vi "Shooter.vi"   [LabVIEW 2012]
uses:
  Robot Global Data.vi
  ShooterStates.ctl
types:
  T1 = typedef "ShooterStates.ctl" = enum16{"Begin", "Spin Wheel", "Window Motor Spin", "Window Motor Wait", "Window Motor Off", "Finish"}
  T2 = typedef "WPI_MotorControlDeviceRef.ctl" = cluster{"DeviceStatus":errorcluster, "Type":enum16{"PWM", "CAN"}, "PWM":cluster{"Digital Module":T3, "PWM Channel":T4, "DeadBand":T5}, "CAN":cluster{"Device Number":u8, "Control Mode":T6, "Semaphore":T7, "Max Vout":dbl}, "Invert":bool, "TransformRef":T8, "InvTransformRef":T8}
  T3 = typedef "FPGA_TypedefDigitalModule.ctl" = enum16{"Digital Module 1", "Digital Module 2"}
  T4 = typedef "FPGA_DIOPWMChannel.ctl" = enum8{"PWM 1", "PWM 2", "PWM 3", "PWM 4", "PWM 5", "PWM 6", "PWM 7", "PWM 8", "PWM 9", "PWM 10", "Invalid"}
  T5 = typedef "WPI_PWMDeadband.ctl" = cluster{"Name":string, "maxPositivePwm":i32, "minPositivePwm":i32, "centerPwm":i32, "maxNegativePwm":i32, "minNegativePwm":i32, "angularRange":u16}
  T6 = typedef "WPI_CANJaguar_ControlMode.ctl" = enum8{"Percent VBus", "Current", "Speed", "Position", "Voltage"}
  T7 = typedef "Semaphore RefNum" = refnum<k1>
  T8 = typedef "WPI_PWMTransform_ConPane.ctl" = refnum<vi>
  T9 = typedef "WPI_JoystickButtonState.ctl" = cluster{"Button 1":bool, "Button 2":bool, "Button 3":bool, "Button 4":bool, "Button 5":bool, "Button 6":bool, "Button 7":bool, "Button 8":bool, "Button 9":bool, "Button 10":bool, "Button 11":bool, "Button 12":bool}
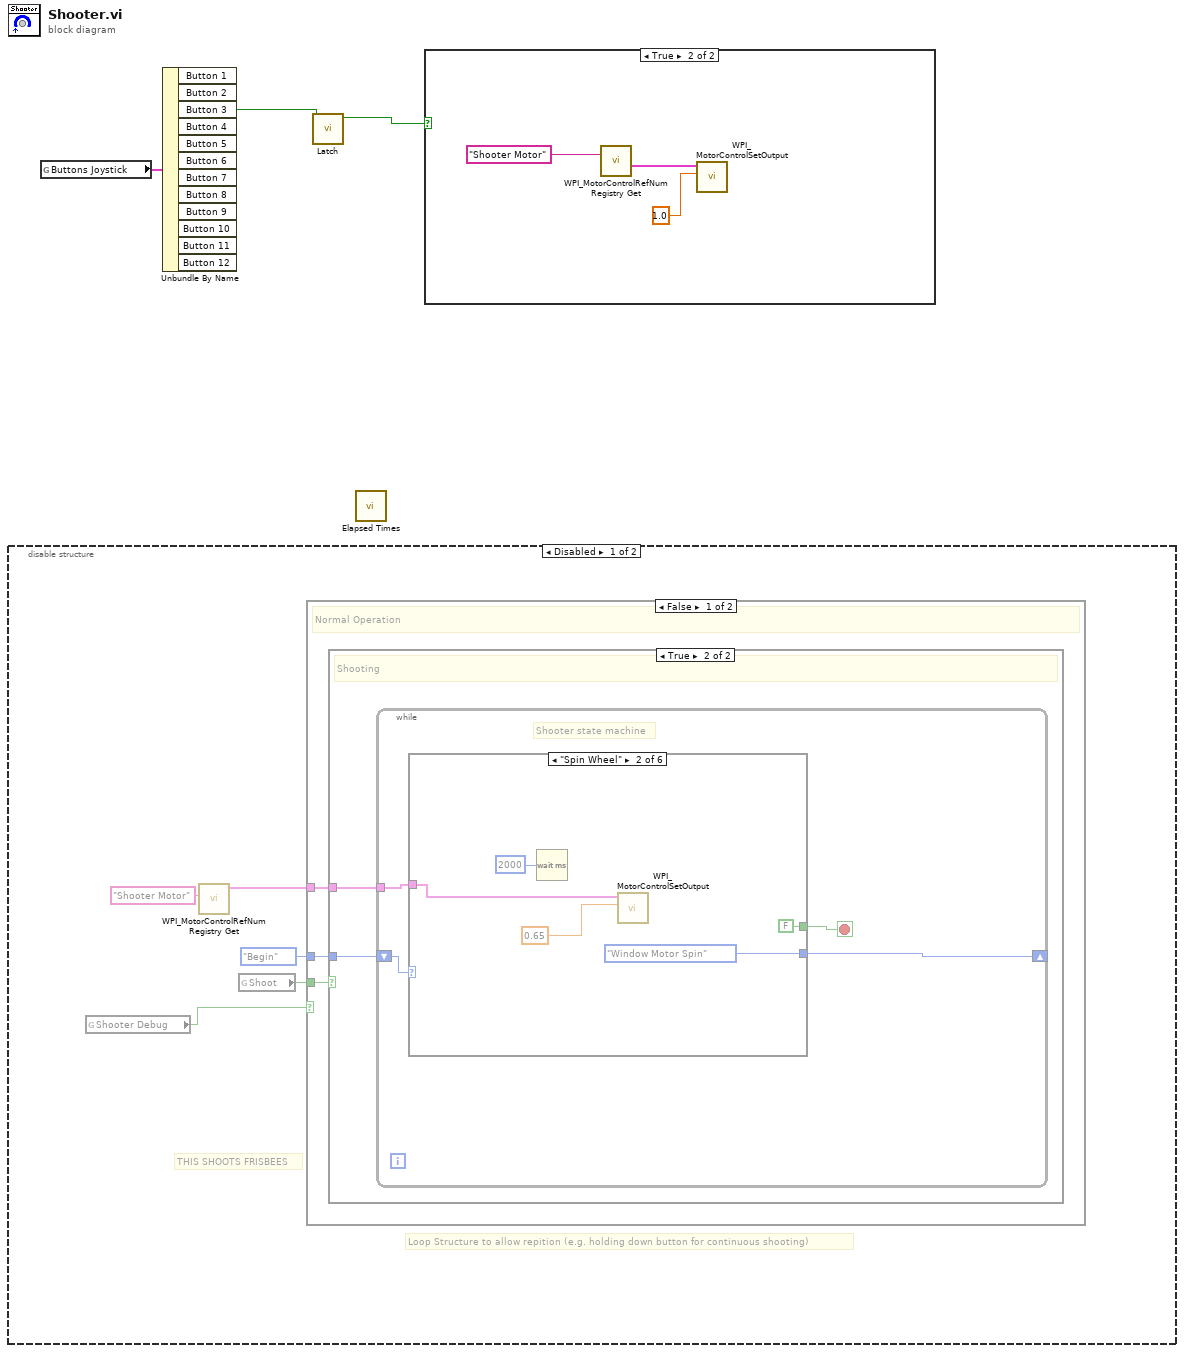
[diagram p0: block diagram]
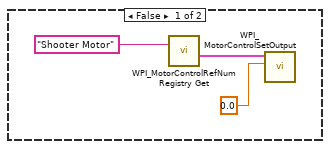
[diagram p2: hidden frame]
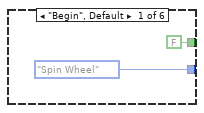
[diagram p4: hidden frame]
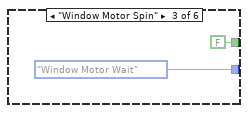
[diagram p5: hidden frame]
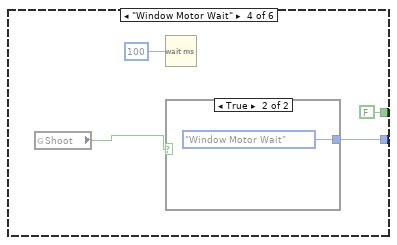
[diagram p6: hidden frame]
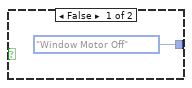
[diagram p7: hidden frame]
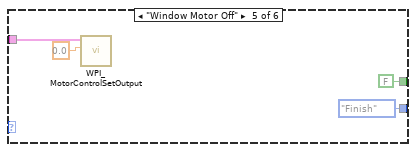
[diagram p8: hidden frame]
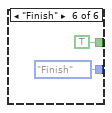
[diagram p9: hidden frame]
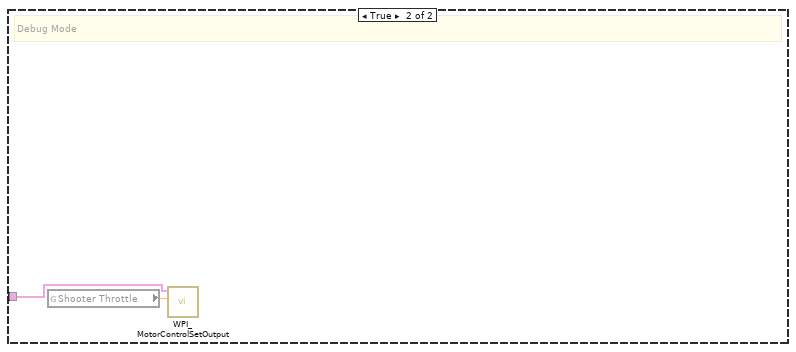
[diagram p10: hidden frame]
diagram:
  n1 = disable-structure shown="Disabled" {
    frame Disabled {
      # "Loop Structure to allow repition (e.g. holding down button for continuous shooting)"
      # "THIS SHOOTS FRISBEES"
      n2 = global read "Robot Global Data.vi" "Shooter Debug"() -> (w4:bool)
      n3 = call <vilib>:"WPI_MotorControlRefNum Registry Get.vi"("refnum name"="Shooter Motor") -> ("MotorControlDevRef"=w5:T2)  [unwired: 9 in, 1 out]
      n4 = global read "Robot Global Data.vi" "Shoot"() -> (w6:bool)
      n5 = case shown="False" w4 {
        tunnel: ShooterStates."Begin" -> [w11 _]
        tunnel: w5 -> [w10 w39]
        tunnel: w6 -> [w9 _]
        frame False {
          # "Normal Operation"
          n6 = case shown="True" w9 {
            tunnel: w11 -> [_ w13]
            tunnel: w10 -> [_ w12]
            frame False {
              # "Not Shooting"
            }
            frame True {
              # "Shooting"
              n7 = while {
                shift-right: [w16] -> _
                shift-left: w13 -> [w17]
                tunnel: w12 -> [w15]
                stop <- w14 stop-if-true
                # "Shooter state machine"
                n8 = case shown="\"Spin Wheel\"" w17 {
                  tunnel: [ShooterStates."Spin Wheel" ShooterStates."Window Motor Spin" ShooterStates."Window Motor Wait" w30 ShooterStates."Finish" ShooterStates."Finish"] -> w16
                  tunnel: w15 -> [_ w21 _ _ w35 _]
                  tunnel: [FALSE FALSE FALSE FALSE FALSE TRUE] -> w14
                  frame "Begin", Default {
                  }
                  frame "Spin Wheel" {
                    n9 = Wait (ms)(milliseconds to wait=u32 2000) -> ()  [unwired: 1 out]
                    n10 = call <vilib>:"WPI_MotorControlSetOutput.vi"("Output"=0.65, "MotorControlDevRef"=w21) -> ()  [unwired: 7 in, 3 out]
                  }
                  frame "Window Motor Spin" {
                  }
                  frame "Window Motor Wait" {
                    n11 = global read "Robot Global Data.vi" "Shoot"() -> (w27:bool)
                    n12 = Wait (ms)(milliseconds to wait=u32 100) -> ()  [unwired: 1 out]
                    n13 = case shown="True" w27 {
                      tunnel: [ShooterStates."Window Motor Off" ShooterStates."Window Motor Wait"] -> w30
                      frame False {
                      }
                      frame True {
                      }
                    }
                  }
                  frame "Window Motor Off" {
                    n14 = call <vilib>:"WPI_MotorControlSetOutput.vi"("Output"=0.0, "MotorControlDevRef"=w35) -> ()  [unwired: 7 in, 3 out]
                  }
                  frame "Finish" {
                  }
                }
              }
            }
          }
        }
        frame True {
          # "Debug Mode"
          n15 = global read "Robot Global Data.vi" "Shooter Throttle"() -> (w40:dbl)
          n16 = call <vilib>:"WPI_MotorControlSetOutput.vi"("Output"=w40, "MotorControlDevRef"=w39) -> ()  [unwired: 7 in, 3 out]
        }
      }
    }
    frame Enabled {
    }
  }
  n17 = global read "Robot Global Data.vi" "Buttons Joystick"() -> (w3:T9)
  n18 = Unbundle By Name(w3) -> ("Button 3"=w2:bool)  [unwired: 11 out]
  n19 = call "Latch.vi"("Input"=w2) -> ("Output"=w1:bool)  [unwired: 9 in]
  n20 = call "Elapsed Times.vi"() -> ()  [unwired: 3 in, 1 out]
  n21 = case shown="True" w1 {
    frame False {
      n22 = call <vilib>:"WPI_MotorControlRefNum Registry Get.vi"("refnum name"="Shooter Motor") -> ("MotorControlDevRef"=w42:T2)  [unwired: 9 in, 1 out]
      n23 = call <vilib>:"WPI_MotorControlSetOutput.vi"("Output"=0.0, "MotorControlDevRef"=w42) -> ()  [unwired: 7 in, 3 out]
    }
    frame True {
      n24 = call <vilib>:"WPI_MotorControlRefNum Registry Get.vi"("refnum name"="Shooter Motor") -> ("MotorControlDevRef"=w45:T2)  [unwired: 9 in, 1 out]
      n25 = call <vilib>:"WPI_MotorControlSetOutput.vi"("Output"=1.0, "MotorControlDevRef"=w45) -> ()  [unwired: 7 in, 3 out]
    }
  }
